vi "KtoC.vi"(11 "K":dbl[](array[numeric])) -> (3 "C":dbl[](array[numeric]))   [LabVIEW 2022 SP3]
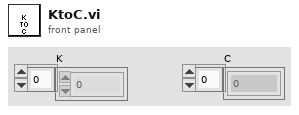
[diagram p1: front panel]
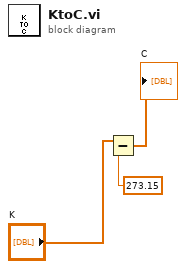
[diagram p0: block diagram]
diagram:
  n1 = Subtract(x="K", y=273.15) -> (x-y=→"C":dbl[])
